vi "Sub VI.vi"() -> ()   [LabVIEW 2010]
panel:
  in  "stop":bool
  # "This is a mock new window"
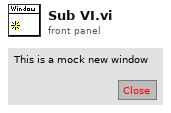
[diagram p1: front panel]
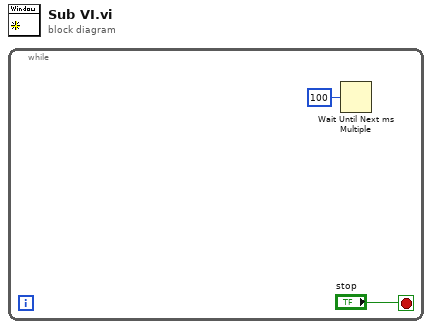
[diagram p0: block diagram]
diagram:
  n1 = while {
    stop <- "stop" stop-if-true
    n2 = Wait Until Next ms Multiple(millisecond multiple=u32 100) -> ()  [unwired: 1 out]
  }
